vi "ROI grp-Remove duplicate ROI indexes.vi"(9 "New POI indexes":i32[](array[numeric]), 11 "Current values in group to be edited":string[](array[string])) -> (1 "No unique new indexes to be added":bool, 3 "New values that do not aldeady exist in the group":string[][](array[string]))   [LabVIEW 2017]
panel:
  out "Number of new unique POI indexes to be added":i32
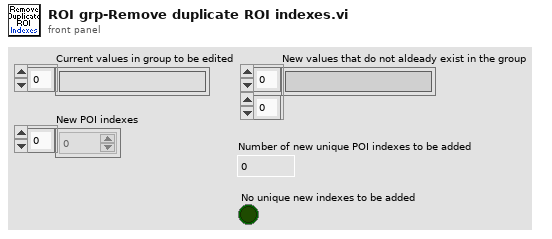
[diagram p1: front panel]
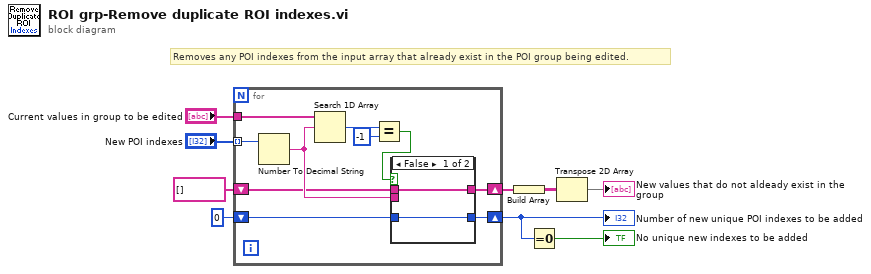
[diagram p0: block diagram]
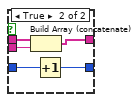
[diagram p2: hidden frame]
diagram:
  # "Removes any POI indexes from the input array that already exist in the POI group being edited."
  n1 = for {
    tunnel: "New POI indexes" -> [w19] mode=indexing
    tunnel: "Current values in group to be edited" -> [w18]
    shift-right: [w13] -> w7
    shift-left: string[] [] -> [w14]
    shift-right: [w10] -> w2
    shift-left: 0 -> [w11]
    n2 = Number To Decimal String(number=w19) -> (decimal integer string=w15:string)  [unwired: 1 in]
    n3 = Search 1D Array(1D array=w18, element=w15) -> (index of element=w17:i32)  [unwired: 1 in]
    n4 = Equal?(x=w17, y=-1) -> (x = y?=w12:bool)
    n5 = case shown="False" w12 {
      tunnel: w15 -> [_ w26]
      tunnel: w14 -> [w21 w25]
      tunnel: [w21 w24] -> w13
      tunnel: w11 -> [w20 w23]
      tunnel: [w20 w22] -> w10
      frame False {
      }
      frame True {
        n6 = Build Array (concatenate)(w25, w26) -> (w24:string[])
        n7 = Increment(x=w23) -> (x+1=w22:i32)
      }
    }
  }
  "Number of new unique POI indexes to be added" <- w2
  n8 = Build Array(w7) -> (w4:string[][])
  n9 = Equal To 0?(x=w2) -> (x = 0?=→"No unique new indexes to be added":bool)
  n10 = Transpose 2D Array(2D array=w4) -> (transposed array=→"New values that do not aldeady exist in the group":string[][])
